vi "Anritsu1b_MT8852B_YYLL_SimpleSet.vi"(11 "YTESTER测试数据":T1) -> (3 "YTESTER结论":T2)   [LabVIEW 2017]
doc: "VIDescription=线损设置"
uses:
  YtCommon.lvlibp/yt`Step StepBaseInput.ctl
  YtCommon.lvlibp/yt`Step StepResult.ctl
  YtCommon.lvlibp/yt`Step TestData.ctl
  YtCommon.lvlibp/yt`Step System Queue.ctl
  YtCommon.lvlibp
panel:
  out "Show":bool
  out "view send":string
  out "read buffer":string
  in  "YTESTER开放参数":T4={"YTESTER_BaseInput"={"isTest"=TRUE, "isSkip"=FALSE, "StepName"="AnritsuMT8852B简单设置", "OnPass"=enum."Next", "OnFail"=enum."Next", "ReTestNumber"=0.0}, "VISA resource name"="", "低频线损dB[-40,0]"=-0.1, "中频线损dB[-40,0]"=-0.1, "高频线损dB[-40,0]"=-0.1, "单隙灵敏度测试-Tx发射功率dBm[-90,0]"=-70.0, "单隙灵敏度测试-包数量[1,10000]"=600}
  # "PathLose & SS \nSimple Set"
  # "MT8852B"
  # "Anritsu"
  # "YYLL"
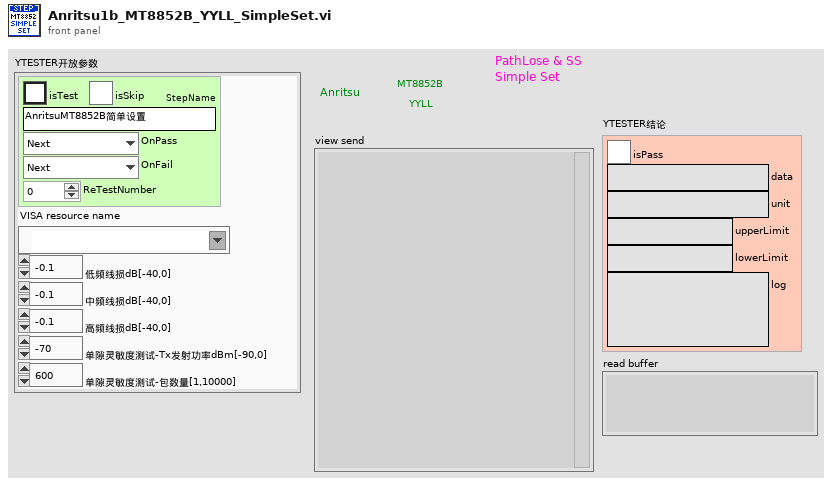
[diagram p1: front panel]
types:
  T1 = typedef "YtCommon.lvlibp/yt`Step TestData.ctl" = cluster{"Socket(From1)":i32, "SN":refnum<notifier>, "StopFlagRef":refnum<notifier>, "YT System Queue":refnum<queue>}
  T2 = typedef "YtCommon.lvlibp/yt`Step StepResult.ctl" = cluster{"isPass":bool, "data":string, "unit":string, "upperLimit":string, "lowerLimit":string, "log":string}
  T3 = typedef "YtCommon.lvlibp/yt`Step StepBaseInput.ctl" = cluster{"isTest":bool, "isSkip":bool, "StepName":string, "OnPass":enum16{"Next", "ToOVER", "Terminate"}, "OnFail":enum16{"Next", "ToOVER", "Terminate"}, "ReTestNumber":dbl}
  T4 = cluster{"YTESTER_BaseInput":T3, "VISA resource name":refnum<visa-resource-name>, "低频线损dB[-40,0]":dbl, "中频线损dB[-40,0]":dbl, "高频线损dB[-40,0]":dbl, "单隙灵敏度测试-Tx发射功率dBm[-90,0]":dbl, "单隙灵敏度测试-包数量[1,10000]":u32}
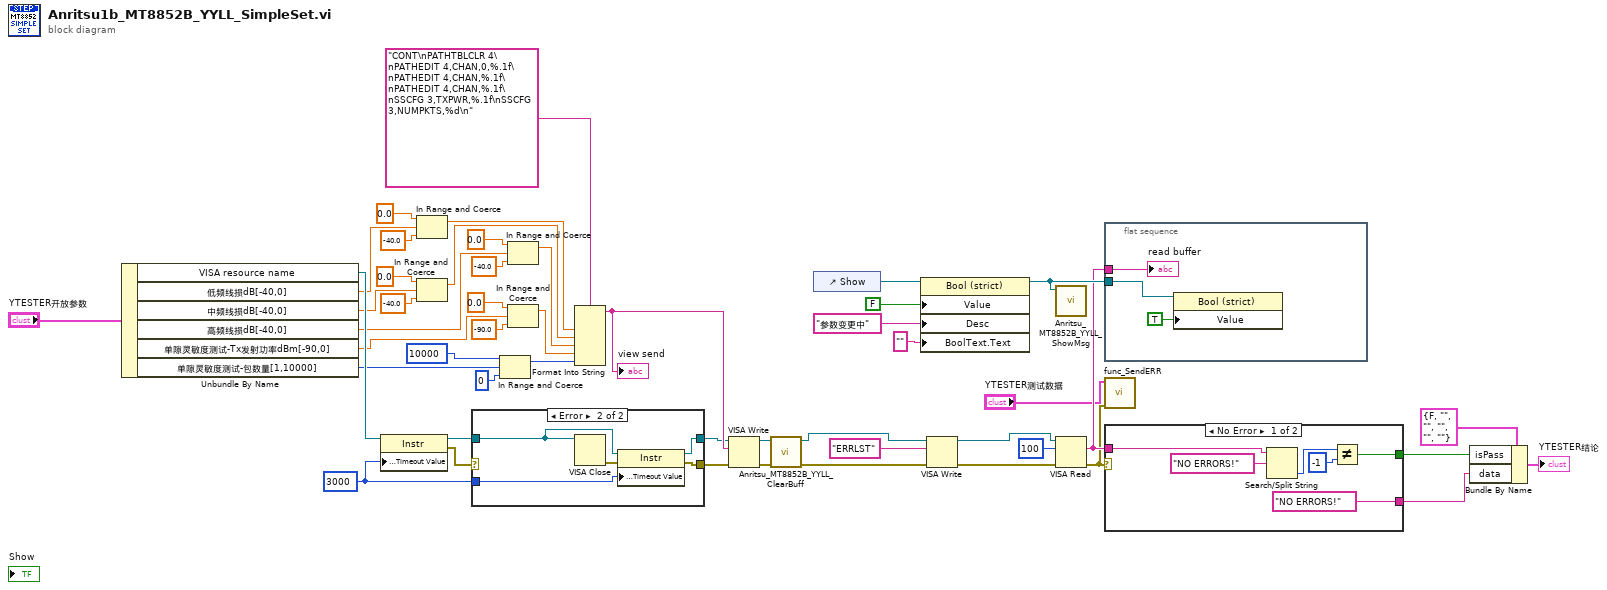
[diagram p0: block diagram]
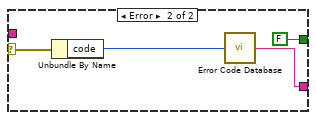
[diagram p3: hidden frame]
diagram:
  w5 = u32 3000 ("General Settings:Timeout Value")
  n1 = Unbundle By Name("YTESTER开放参数") -> ("VISA resource name"=w38:refnum<visa-resource-name>, "低频线损dB[-40,0]"=w31:dbl, "中频线损dB[-40,0]"=w30:dbl, "高频线损dB[-40,0]"=w29:dbl, "单隙灵敏度测试-Tx发射功率dBm[-90,0]"=w21:dbl, "单隙灵敏度测试-包数量[1,10000]"=w18:u32)
  n2 = property class="Instr"(reference=w38, "General Settings:Timeout Value"=w5) -> (reference out=w6:refnum<visa-resource-name>, error out=w7:errorcluster)  [unwired: 1 in]
  n3 = In Range and Coerce(upper limit=0.0, x=w31, lower limit=-40.0) -> (coerced(x)=w27:dbl)  [unwired: 1 out]
  n4 = In Range and Coerce(upper limit=0.0, x=w30, lower limit=-40.0) -> (coerced(x)=w26:dbl)  [unwired: 1 out]
  n5 = case shown="Error" w7 {
    selector: w7 -> [w50 _]
    tunnel: w6 -> [w51 w56]
    tunnel: w5 -> [_ w54]
    tunnel: [w50 w53] -> w4
    tunnel: [w51 w52] -> w3
    frame No Error {
    }
    frame Error {
      n6 = VISA Close(VISA resource name=w56) -> (error out=w55:errorcluster)  [unwired: 1 in]
      n7 = property class="Instr"(reference=w56, error in=w55, "General Settings:Timeout Value"=w54) -> (reference out=w52:refnum<visa-resource-name>, error out=w53:errorcluster)
    }
  }
  n8 = In Range and Coerce(upper limit=u32 10000, x=w18, lower limit=u32 0) -> (coerced(x)=w8:u32)  [unwired: 1 out]
  n9 = In Range and Coerce(upper limit=0.0, x=w29, lower limit=-40.0) -> (coerced(x)=w25:dbl)  [unwired: 1 out]
  n10 = In Range and Coerce(upper limit=0.0, x=w21, lower limit=-90.0) -> (coerced(x)=w9:dbl)  [unwired: 1 out]
  n11 = Format Into String(format string="CONT\nPATHTBLCLR 4\nPATHEDIT 4,CHAN,0,%.1f\nPATHEDIT 4,CHAN,%.1f\nPATHEDIT 4,CHAN,%.1f\nSSCFG 3,TXPWR,%.1f\nSSCFG 3,NUMPKTS,%d\n", w27, w26, w25, w9, w8) -> (resulting string=w24:string)  [unwired: 2 in, 1 out]
  "view send" <- w24
  n12 = VISA Write(VISA resource name=w3, write buffer=w24, error in (no error)=w4) -> (VISA resource name out=w43:refnum<visa-resource-name>, error out=w41:errorcluster)  [unwired: 1 out]
  n13 = call "Anritsu_MT8852B_YYLL_ClearBuff.vi"("error IO"=w41, "VISA resource name"=w43) -> ("error IO 2"=w40:errorcluster, "VISA resource name 2"=w42:refnum<visa-resource-name>)  [unwired: 7 in, 1 out]
  n14 = control-ref of="Show"() -> (w16:refnum<vi>)
  n15 = property on="Property Node" class="Bool (strict)"(reference=w16, "Value"=FALSE, "Desc"="参数变更中" ("String"), "BoolText.Text"="" ("Boolean Text.Text")) -> (reference out=w14:refnum<vi>)  [unwired: 1 in, 1 out]
  n16 = VISA Write(VISA resource name=w42, write buffer="ERRLST", error in (no error)=w40) -> (VISA resource name out=w45:refnum<visa-resource-name>, error out=w44:errorcluster)  [unwired: 1 out]
  n17 = call "Anritsu_MT8852B_YYLL_ShowMsg.vi"("reference out"=w14) -> ()  [unwired: 11 in]
  n18 = VISA Read(VISA resource name=w45, byte count=u32 100 ("byte count (0)"), error in (no error)=w44) -> (read buffer=w13:string, error out=w11:errorcluster)  [unwired: 2 out]
  n19 = flat-sequence {
    tunnel: w14 -> [w58]
    tunnel: w13 -> [w57]
    frame #0 {
      n20 = property on="Property Node" class="Bool (strict)"(reference=w58, "Value"=TRUE) -> ()  [unwired: 1 in, 2 out]
      "read buffer" <- w57
    }
  }
  n21 = call "func_SendERR.vi"("ERR (String\\Errclust)"=w11, "YTESTER测试数据 in"="YTESTER测试数据") -> ()  [unwired: 9 in, 1 out]
  n22 = case shown="No Error" w11 {
    selector: w11 -> [_ w68]
    tunnel: [w61 FALSE] -> w17
    tunnel: w13 -> [w62 _]
    tunnel: ["NO ERRORS!" ("search string/char (-)") w66] -> w10
    frame No Error {
      n23 = Search/Split String(string=w62, search string/char (-)="NO ERRORS!") -> (offset of match=w65:i32)  [unwired: 1 in, 2 out]
      n24 = Not Equal?(x=w65, y=-1) -> (x != y?=w61:bool)
    }
    frame Error {
      n25 = Unbundle By Name(w68) -> ("code"=w67:i32)
      n26 = call <vilib>:"Error Code Database.vi"("Error Code"=w67) -> ("Error Text"=w66:string)
    }
  }
  n27 = Bundle By Name(cluster=T2 {"isPass"=FALSE, "data"="", "unit"="", "upperLimit"="", "lowerLimit"="", "log"=""} ("Result"), "isPass"=w17, "data"=w10) -> (→"YTESTER结论":T2)
